vi "FaulhaberV3-Ascii.vi"() -> ()   [LabVIEW 2011]
panel:
  out "Kommentar":string[](array[string])
  out "Default":i32[](array[numeric])
  out "rw":enum16{"unknown", "ro", "rw", "wo", "const"}[](array[ring])
  out "Name":string[](array[string])
  out "Typ":T1(array[ring])
  out "ID-16.08":u32[](array[numeric]) format="%x"
  out "String 1":string
  in  "?":string="0x2313.01\tR32\tAIn1Gain\trw\t2147450880\tAnalogGain\n0x2313.02\tS16\tAIn1Offset\trw\t-2500\tAnalogOffset\n0x2313.09\tS16\tAIn1VirtualValue\trw\t0\tAnalogSimulieren\n0x2313.0A\tU8\tAIn1EnableVirtual\trw\t0\tSimulierten wert nehmen\n0x2324.01\tU32\tStatus\tro\t0\tGerätezustandwort: 0Speed,1TargetSpeedReached,2WrongSpeed,3TargetPosReached, 4PsoSoll, 5Outofcorridor, 6PosLimitswitch,7NegLimitSwitch, 8PosSowratelimit,9NegSoftware, 10Ref, 11Encoder, 12Referenziert, 13Vlimit,14TLimit,15VLimit,16TempWarn,17TempOut, 18Vcchigh, 19VccLow, 20VMotLow, 21Speederr, 24..31 DigIn1..8\n0x2331.00\tU8\tEntriesTagetSource\tro\t4\tTagetSourceEtries\n0x2331.01\tU8\tTargetVoltageSource\trw\t0\tTargetVoltageSource\n0x2331.02\tU8\tTargetCurrentSource\trw\t0\tTargetCurrentSource\n0x2331.03\tU8\tTargetVelSource\trw\t0\tTargetVelSource\n0x2331.04\tU8\tTargetPosSource\trw\t0\tAnalogIn1=1, AnalogIn2=2\n0x6040.00\tU16\tControl\trw\t0\tBit0=,B4=NewSetpoint,B5=ChangeImmediately,B6=rel, B9=keinAbbremsen, \n0x6041.00\tU16\tGSW\tro\tNaN\tStatusword\n0x6060.00\tS8\tModus\trw\t0\t0=aus, 1=PP\n0x6060.00\tS8\tModeOperation\trw\t0\tCommunikationssystem 1:PP, 3PV, 0:aus, -2= analog?, -3=AnalogSpeed, -4=AnalogTorque, 6Homing\n0x6062.00\tS32\tPositionDemandValue\tro\tNaN\tSollposiitonlesen?\n0x6064.00\tS32\tPOS\tro\tNaN\tIstposition lesen\n0x6078.00\tS16\tGRC\tro\t0\tAktueller Strom\n0x607A.00\tS32\tTargetPosition\trw\t0\tZielposition setzen\n0x6081.00\tU32\tProfileVel\trw\t32767\tProfil Geschwindigkeit\n0x6083.00\tU32\tPorfileAcc\trw\t30000\tProfil Beschleunigung\n0x6084.00\tU32\tProfileDec\trw\t30000\tProil Bremsen\n0x6085.00\tU32\tQuickstop\trw\t30000\tQuickstop deceleration\n0x6086.00\tS16\tProfileType\trw\t0\tTyp0=linear, 1=Sin^2\n0x60E0.00\tU16\tPosTorqueLimit\trw\t6000\t1000=100%=Nennmoment\n0x60E1.00\tU16\tNegTorqueLimit\trw\t6000\t1000=100%=Nennmoment\n0x608F.00\tU8\tEntriesPosEncoder\tro\t2\tEncoderEntries\n0x608F.01\tU32\tPosEncoderIncrements\tro\t4096\tEncoderincremente\n0x608F.02\tU32\tPosMotorRevolutions\tro\t1\tMotordrehungen\n0x6090.00\tU8\tEntriesVelEncoder\tro\t2\tSpeedenecoderEntries\n0x6090.01\tU32\tVelEncoderIncrements\tro\t4096\tAuflösung des Sensors\n0x6090.02\tU32\tVelMotorRevolutions\tro\t1\tMotordrehungen bei 01 genannten Pulsen\n0x6096.00\tS8\tHomingMethod\trw\t0\tHoming Methods\n0x60B0.00\tS32\tPositionOffset\trw\t0\tPosition Offset\n0x60C5.00\tU32\tMaximumAcceleration\trw\t30000\tMaximale beschleunigung PP PV\n0x60C6.00\tU32\tMaximumDeceleration\trw\t30000\tMaximales Bremsen PP PV\n0x60F4.00\tU32\tFollowingErrorActualValue\tro\t0\tAbweichung Soll Ist\n0x60FD.00\tU32\tDigitalInputs\tro\tNan\tBit2: Refinput, Bit 16..32 Digin1..Digin8\n0x60FF.00\tS32 \tTargetVelocity\trw\t0\tgeschwindigkeitssoll\n0x6502.00\tU32\tSupportedDriveModes\tro\tNan\tCia402 Modi\n"
  # "tabs"
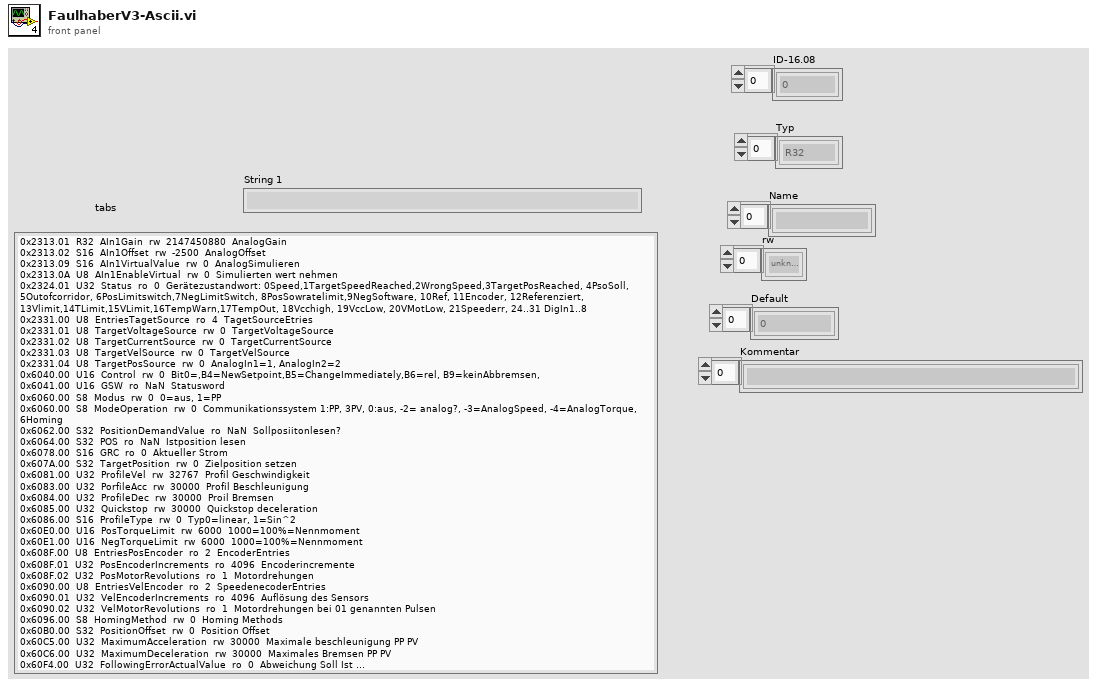
[diagram p1: front panel]
types:
  T1 = enum8{"unknown", "none", "U8", "S8", "U16", "S16", "U32", "S32", "R32", "somethingelse16"}[]
  T2 = enum8{"unknown", "none", "U8", "S8", "U16", "S16", "U32", "S32", "R32", "somethingelse16"}
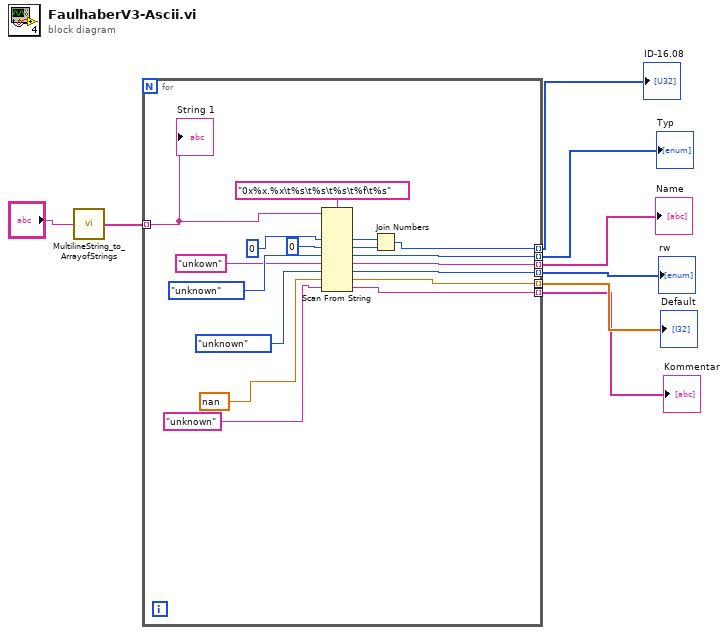
[diagram p0: block diagram]
diagram:
  n1 = call "MultilineString_to_ArrayofStrings.vi"("String 1"="?") -> ("String Array"=w7:string[])  [unwired: 1 in]
  n2 = for {
    tunnel: w7 -> [w25] mode=indexing
    tunnel: [w9] -> w6 mode=indexing
    tunnel: [w18] -> w5 mode=indexing
    tunnel: [w17] -> w4 mode=indexing
    tunnel: [w16] -> w2 mode=indexing
    tunnel: [w15] -> w3 mode=indexing
    tunnel: [w14] -> w1 mode=indexing
    n3 = Scan From String(format string="0x%x.%x\t%s\t%s\t%s\t%f\t%s", input string=w25, default 1=u16 0 ("ID"), default 2=u8 0 ("default value 2"), default 3=T2."unknown" ("Data"), default 4="unkown" ("Name"), default 5=enum16{"unknown", "ro", "rw", "wo", "const"}."unknown" ("Attr"), default 6=nan ("Default"), default 7="unknown" ("Description")) -> (output 1=w11:u16, output 2=w10:u8, output 3=w18:T2, output 4=w17:string, output 5=w15:enum16{"unknown", "ro", "rw", "wo", "const"}, output 6=w16:dbl, output 7=w14:string)  [unwired: 2 in, 3 out]
    n4 = Join Numbers(hi=w11, lo=w10) -> ((hi.lo)=w9:u32)
    "String 1" <- w25
  }
  "ID-16.08" <- w6
  "Typ" <- w5
  "Name" <- w4
  "rw" <- w3
  "Default" <- w2
  "Kommentar" <- w1
